vi "JLink Flash Programming.vi"(7 "Flash Programming Command Type":T1, 8 "error in (no error)":errorcluster, 9 "Flash Programming Configuration":T2={"Erase Configuration"={"Start Address"="", "End Address"="", "Reset"=TRUE}, "LoadFile Configuration"={"File Name"=path "", "Address"="", "Reset"=TRUE}}, 10 "Target Configuration":T3, 11 "JLink Directory":path caption="(Example: C:\\Program Files\\SEGGER\\JLink)") -> (0 "error out":errorcluster, 1 "PASS":bool, 2 "standard output":string)   [LabVIEW 2016, in "JLink Commander.lvlib"]
doc: "This VI performs Flash Programming through JLink Commander."
uses:
  JLink Commander.lvlib
  Type Definitions/Target Configuration.ctl
  Type Definitions/Flash Programming Configuration.ctl
  Type Definitions/Flash Programming Command Type.ctl
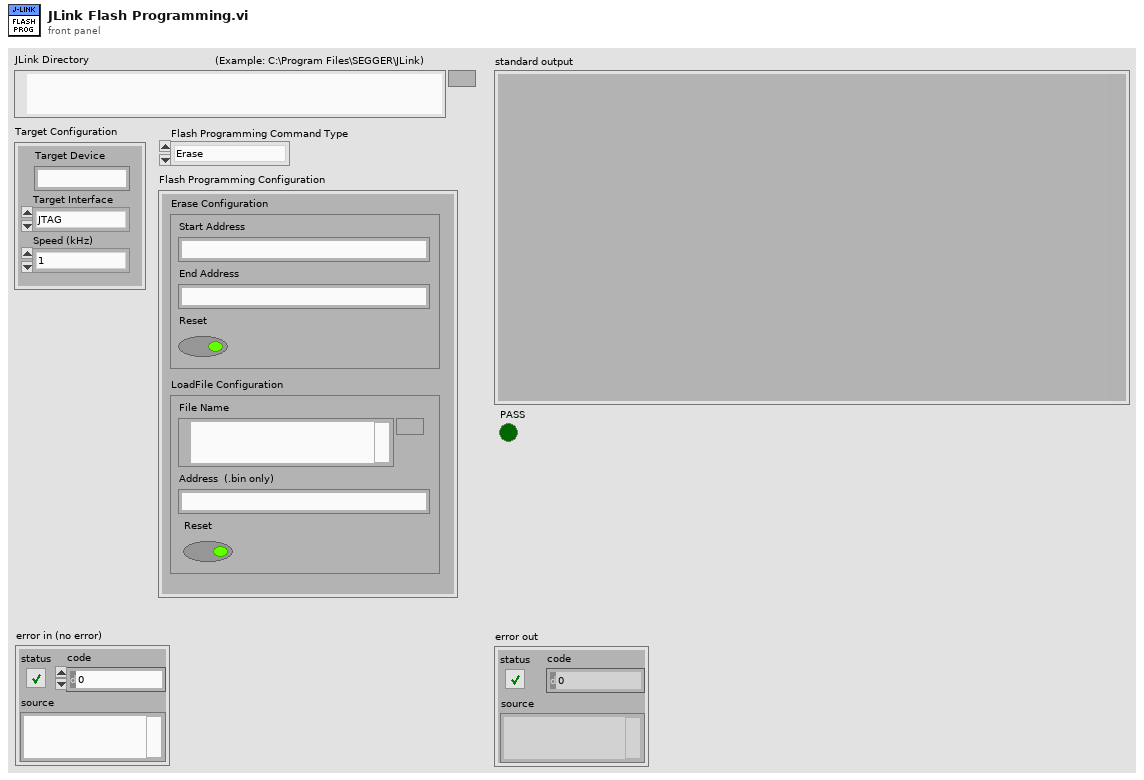
[diagram p1: front panel]
types:
  T1 = typedef "JLink Commander.lvlib/Flash Programming Command Type.ctl" = enum16{"Erase", "ReadBinary", "LoadFile", "SaveBin", "VerifyBin"}
  T2 = typedef "JLink Commander.lvlib/Flash Programming Configuration.ctl" = cluster{"Erase Configuration":cluster{"Start Address":string, "End Address":string, "Reset":bool}, "LoadFile Configuration":cluster{"File Name":path, "Address":string, "Reset":bool}}
  T3 = typedef "JLink Commander.lvlib/Target Configuration.ctl" = cluster{"Target Device":string, "Target Interface":enum16{"JTAG", "SWD", "FINE", "ICSP", "C2", "CJTAG"}, "Speed (kHz)":enum16{"1", "5", "10", "20", "30", "50", "100", "200", "300", "400", "500", "600", "750", "900", "1000", "1334", "1600", "2000", "2667", "3200", "4000", "4800", "5334", "6000", "8000", "9600", "12000", "15000", "20000", "25000", "30000", "40000", "50000"}}
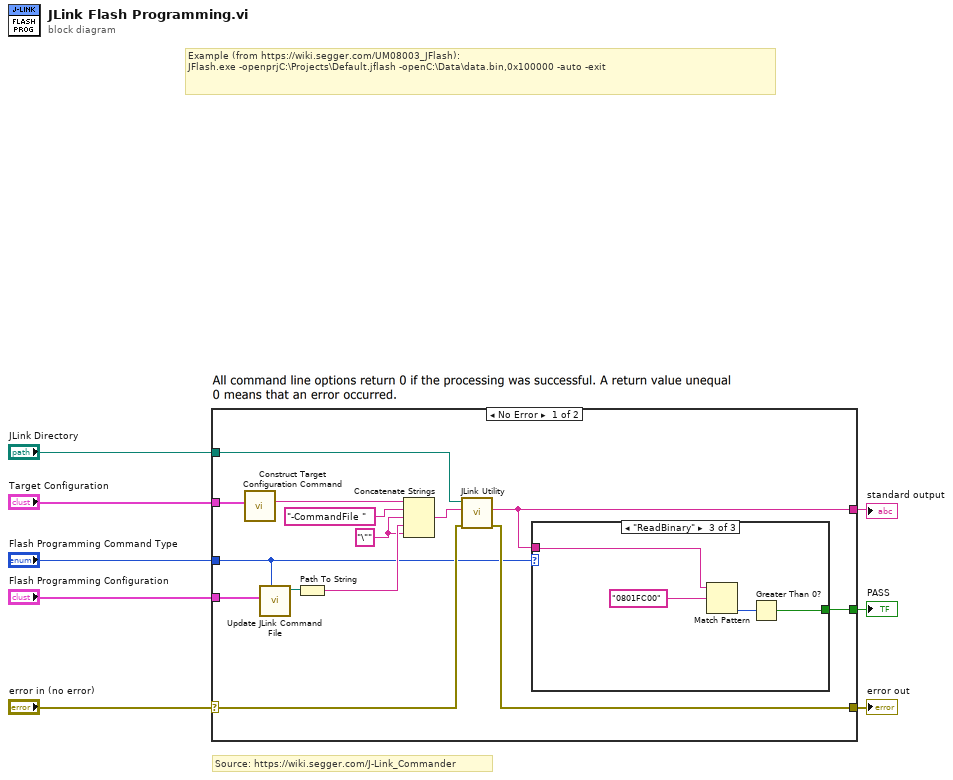
[diagram p0: block diagram]
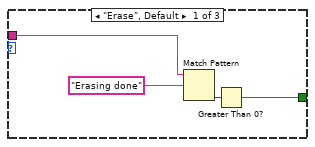
[diagram p2: hidden frame]
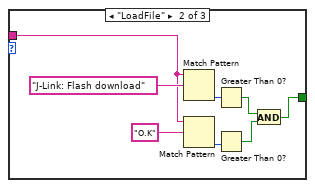
[diagram p3: hidden frame]
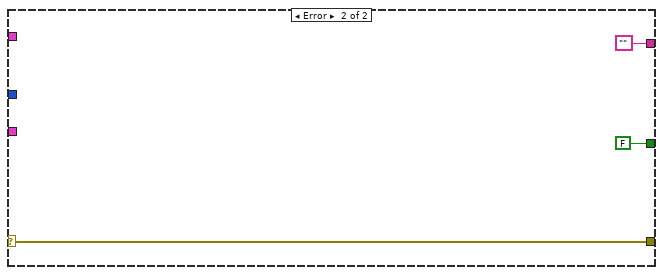
[diagram p4: hidden frame]
diagram:
  # "Source: https://wiki.segger.com/J-Link_Commander"
  # "Example (from https://wiki.segger.com/UM08003_JFlash):\nJFlash.exe -openprjC:\\Projects\\Default.jflash -openC:\\Data\\data.bin,0x100000 -auto -exit"
  n1 = case shown="No Error" "error in (no error)" {
    selector: "error in (no error)" -> [w22 w41]
    tunnel: [w21 w41] -> w7
    tunnel: "JLink Directory" -> [w15 _]
    tunnel: [w12 ""] -> w6
    tunnel: "Target Configuration" -> [w20 _]
    tunnel: "Flash Programming Command Type" -> [w13 _]
    tunnel: "Flash Programming Configuration" -> [w14 _]
    tunnel: [w11 FALSE] -> w1
    frame No Error {
      w9 = "\""
      n2 = call "Construct Target Configuration Command.vi"("Target Configuration"=w20) -> ("Target Configuration Command"=w19:string)  [unwired: 9 in, 1 out]
      n3 = call "Update JLink Command File.vi"("Flash Programming Command Type"=w13, "Flash Programming Configuration"=w14) -> ("J-Link Command File"=w18:path)  [unwired: 7 in, 2 out]
      n4 = Path To String(path=w18) -> (string=w17:string)
      n5 = Concatenate Strings(w19, "-CommandFile ", w9, w17, w9) -> (w16:string)
      n6 = call "JLink Utility.vi"("error in (no error)"=w22, "Parameters String"=w16, "JLink Directory"=w15) -> ("error out"=w21:errorcluster, "standard output"=w12:string)  [unwired: 7 in]
      n7 = case shown="\"ReadBinary\"" w13 {
        tunnel: w12 -> [w26 w27 w35]
        tunnel: [w23 w28 w36] -> w11
        frame "Erase", Default {
          n8 = Match Pattern(string=w26, regular expression="Erasing done" ("string")) -> (offset past match=w24:i32)  [unwired: 1 in, 3 out]
          n9 = Greater Than 0?(x=w24) -> (x > 0?=w23:bool)
        }
        frame "LoadFile" {
          n10 = Match Pattern(string=w27, regular expression="J-Link: Flash download" ("string")) -> (offset past match=w33:i32)  [unwired: 1 in, 3 out]
          n11 = Match Pattern(string=w27, regular expression="O.K" ("string")) -> (offset past match=w31:i32)  [unwired: 1 in, 3 out]
          n12 = Greater Than 0?(x=w33) -> (x > 0?=w30:bool)
          n13 = Greater Than 0?(x=w31) -> (x > 0?=w29:bool)
          n14 = And(x=w30, y=w29) -> (x .and. y?=w28:bool)
        }
        frame "ReadBinary" {
          n15 = Match Pattern(string=w35, regular expression="0801FC00" ("string")) -> (offset past match=w37:i32)  [unwired: 1 in, 3 out]
          n16 = Greater Than 0?(x=w37) -> (x > 0?=w36:bool)
        }
      }
    }
    frame Error {
    }
  }
  "error out" <- w7
  "standard output" <- w6
  "PASS" <- w1
